vi "pf_Find_Port_Number.vi"(8 "error in (no error)":errorcluster, 9 "Port Name":string, 10 "Port Info array":T1[](array[typedef])) -> (0 "error out":errorcluster, 1 "Port Number found":i32, 2 "Port Info found":T1={"Port Number"=-1, "Manufacturer Name"="", "Port Name"="", "CLALLSERIAL Version"=enum."Undefined", "Port Type"=enum."Undefined"})   [LabVIEW 2025, in "Photonfocus_Toolkit.lvlib"]
uses:
  Photonfocus_Toolkit.lvlib
  _Private/Controls/pf_Port_Info.ctl
  _Private/Controls/pf_CLALLSERIAL_Version.ctl
  _Private/Controls/pf_Port_Type.ctl
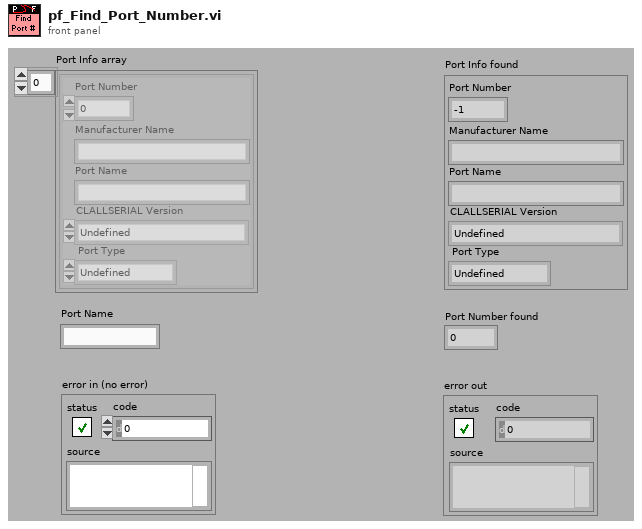
[diagram p1: front panel]
types:
  T1 = typedef "Photonfocus_Toolkit.lvlib/pf_Port_Info.ctl" = cluster{"Port Number":i32, "Manufacturer Name":string, "Port Name":string, "CLALLSERIAL Version":T2, "Port Type":T3}
  T2 = typedef "Photonfocus_Toolkit.lvlib/pf_CLALLSERIAL_Version.ctl" = enum16{"Undefined", "No CLALLSERIAL port", "CL_DLL_VERSION_NO_VERSION", "CL_DLL_VERSION_1_0", "CL_DLL_VERSION_1_1"}
  T3 = typedef "Photonfocus_Toolkit.lvlib/pf_Port_Type.ctl" = enum16{"Undefined", "CLALLSERIAL port", "port with clser.dll", "USB port", "RS-232 port"}
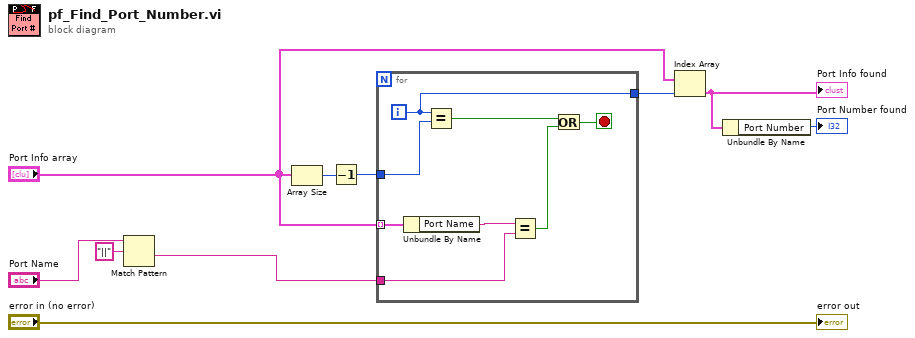
[diagram p0: block diagram]
diagram:
  n1 = Match Pattern(string="Port Name", regular expression="||") -> (after substring=w1:string)  [unwired: 4 out]
  n2 = Array Size(array="Port Info array") -> (size(s)=w10:i32)
  n3 = Decrement(x=w10) -> (x-1=w9:i32)
  n4 = for {
    tunnel: "Port Info array" -> [w18] mode=indexing
    tunnel: w1 -> [w16]
    tunnel: w9 -> [w15]
    tunnel: [w12] -> w8
    i -> [w12]
    stop <- w11 stop-if-true
    n5 = Unbundle By Name(w18) -> ("Port Name"=w17:string)
    n6 = Equal?(x=w12, y=w15) -> (x = y?=w14:bool)
    n7 = Equal?(x=w17, y=w16) -> (x = y?=w13:bool)
    n8 = Or(x=w14, y=w13) -> (x .or. y?=w11:bool)
  }
  n9 = Index Array(array="Port Info array", index=w8) -> (element=w6:T1)
  "Port Info found" <- w6
  n10 = Unbundle By Name(w6) -> ("Port Number"=→"Port Number found":i32)
  "error out" <- "error in (no error)"
